vi "Disassemble message.vi"(8 "error in (no error)":errorcluster, 11 "RxTx in":refnum<class "RxTx.lvclass">) -> (0 "error out":errorcluster, 2 "Message":string, 3 "RxTx out":refnum<class "RxTx.lvclass">)   [LabVIEW 2012, in "RxTx.lvclass"]
uses:
  RxTx.lvclass
  RxTx.lvclass/RxTx.ctl
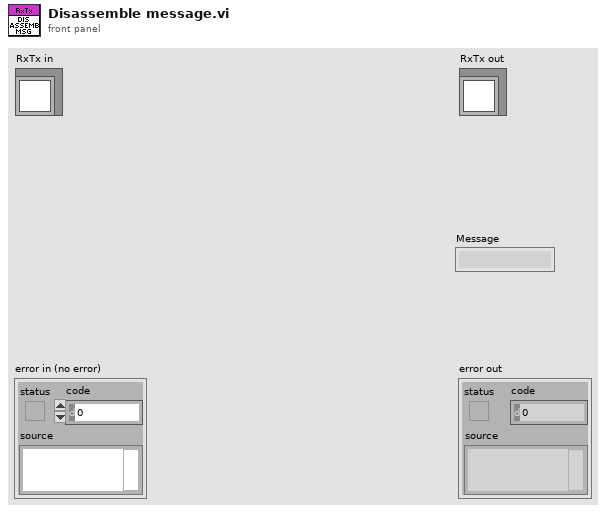
[diagram p1: front panel]
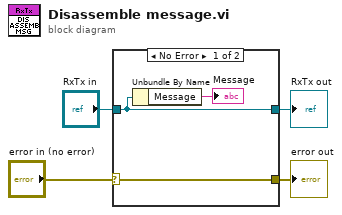
[diagram p0: block diagram]
diagram:
  n1 = case shown="No Error" "error in (no error)" {
    selector: "error in (no error)" -> [w7 w9]
    tunnel: [w7 w9] -> w3
    tunnel: [w6 w8] -> w1
    tunnel: "RxTx in" -> [w6 w8]
    frame No Error {
      n2 = Unbundle By Name(w6) -> ("Message"=→"Message":string)
    }
    frame Error {
    }
  }
  "error out" <- w3
  "RxTx out" <- w1
